vi "Activate-hardware.vi"(8 "error in (no error)":errorcluster, 11 "Data ref. in":refnum<data-value>) -> (0 "error out":errorcluster, 1 "Succes?":bool, 3 "Data ref.":refnum<data-value>)   [LabVIEW 2013, in "CameraVision.lvlib" / "CV-Main.lvclass"]
uses:
  CV-Main.lvclass
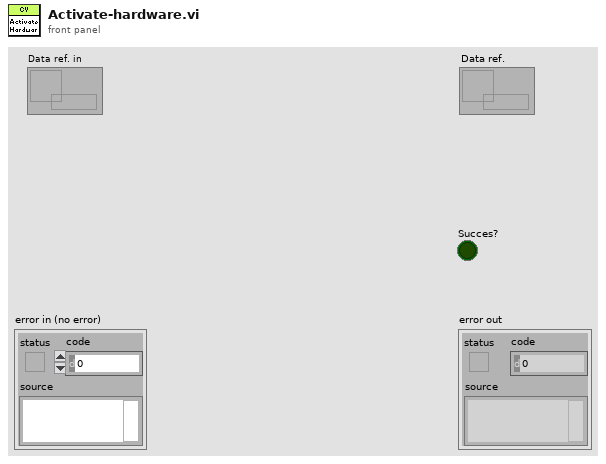
[diagram p1: front panel]
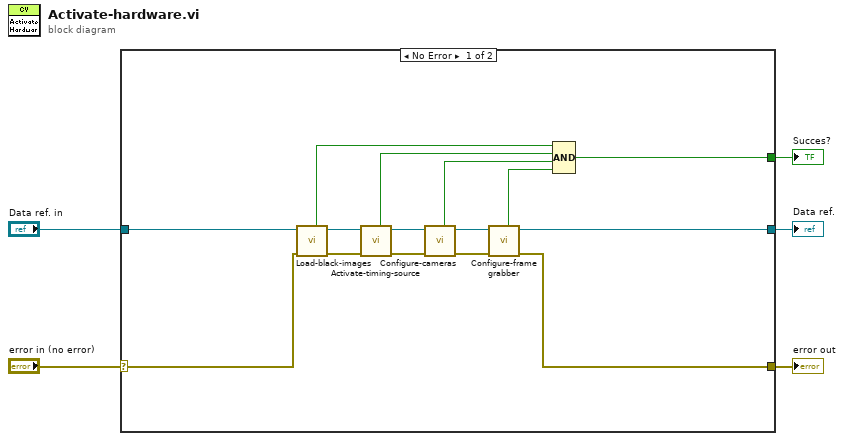
[diagram p0: block diagram]
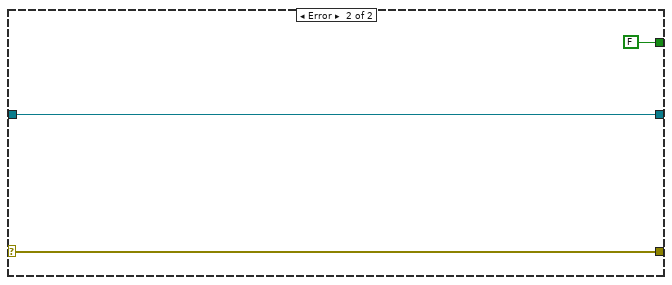
[diagram p2: hidden frame]
diagram:
  n1 = case shown="No Error" "error in (no error)" {
    selector: "error in (no error)" -> [w11 w23]
    tunnel: [w9 w23] -> w4
    tunnel: "Data ref. in" -> [w12 w22]
    tunnel: [w14 w22] -> w2
    tunnel: [w15 FALSE] -> w1
    frame No Error {
      n2 = call "Load-black-images.vi"("error in"=w11, "Data ref. in"=w12) -> ("error IO"=w8:errorcluster, "Data ref."=w13:refnum<data-value>, "Success?"=w10:bool)  [unwired: 7 in]
      n3 = call "Activate-timing-source.vi"("error in"=w8, "Data ref. in"=w13) -> ("error IO"=w6:errorcluster, "Data ref."=w7:refnum<data-value>, "Succes?"=w19:bool)  [unwired: 7 in]
      n4 = call "Configure-cameras.vi"("error in"=w6, "Data ref. in"=w7) -> ("error IO"=w18:errorcluster, "Data ref."=w16:refnum<data-value>, "Succes?"=w20:bool)  [unwired: 6 in, 1 out]
      n5 = call "Configure-framegrabber.vi"("error in"=w18, "Data ref. in"=w16) -> ("error IO"=w9:errorcluster, "Data ref."=w14:refnum<data-value>, "Succes?"=w17:bool)  [unwired: 6 in, 1 out]
      n6 = Compound Arithmetic op=AND(w10, w19, w20, w17) -> (w15:bool)
    }
    frame Error {
    }
  }
  "error out" <- w4
  "Data ref." <- w2
  "Succes?" <- w1
